vi "_Parse Segment Limit Check Array Result.vi"(8 "error in (no error)":errorcluster, 10 "Input String":string, 11 "VISA resource name":refnum<visa-resource-name>) -> (0 "error out":errorcluster, 1 "Results":i32[](array[numeric]), 2 "Reliability Results":T1, 3 "VISA resource name out":refnum<visa-resource-name>, 5 "Out Of Tolerance":dbl format="%^.3e", 7 "Statistic Expired":i32)   [LabVIEW 2020, in "Rohde&Schwarz CMXP NR FR2 Measurement.lvlib"]
uses:
  <instrlib>/Rohde&Schwarz CMXP NR FR2 Measurement/Rohde&Schwarz CMXP NR FR2 Measurement.lvlib
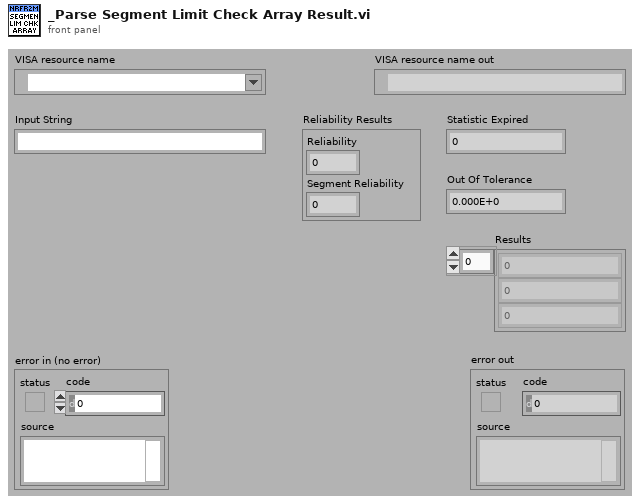
[diagram p1: front panel]
types:
  T1 = cluster{"Reliability":i32, "Segment Reliability":i32}
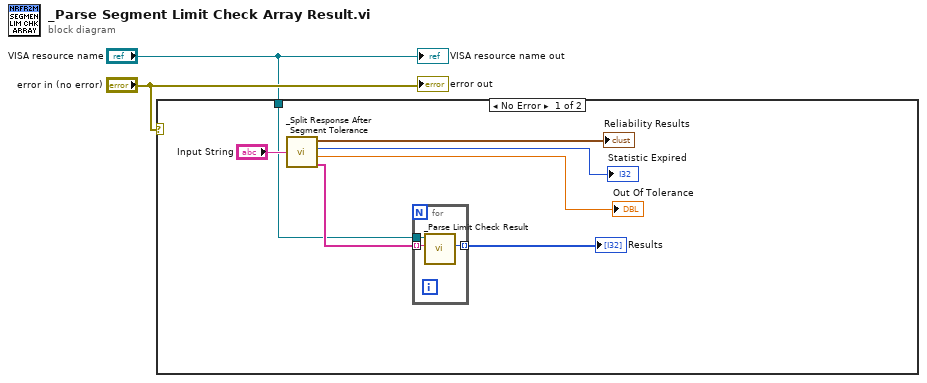
[diagram p0: block diagram]
diagram:
  n1 = case shown="No Error" "error in (no error)" {
    tunnel: "VISA resource name" -> [w3 _]
    frame No Error {
      n2 = call <instrlib>:"_Split Response After Segment Tolerance.vi"("Input String"="Input String") -> ("Reliability Results"=→"Reliability Results":T1, "Statistic Expired"=→"Statistic Expired":i32, "Out Of Tolerance"=→"Out Of Tolerance":dbl, "Response out"=w5:string[])
      n3 = for {
        tunnel: w5 -> [w12] mode=indexing
        tunnel: [w11] -> w4 mode=indexing
        tunnel: w3 -> [w10]
        n4 = call <instrlib>:"_Parse Limit Check Result.vi"("String Value In"=w12, "VISA resource name"=w10) -> ("Limit Check Value"=w11:i32)  [unwired: 7 in, 2 out]
      }
      "Results" <- w4
    }
    frame Error {
    }
  }
  "VISA resource name out" <- "VISA resource name"
  "error out" <- "error in (no error)"
